vi "SP SP - get ctrl.vi"(8 "error in (no error)":errorcluster, 10 "subpanel":string, 11 "subsubpanel":string) -> (0 "error out":errorcluster, 2 "Boolean":bool, 3 "VI out":refnum<vi>)   [LabVIEW 2020, in "ui-testing.lvlib"]
uses:
  ui-testing.lvlib
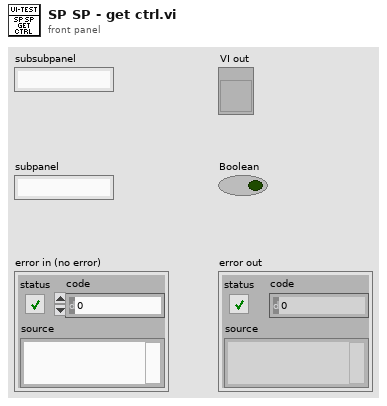
[diagram p1: front panel]
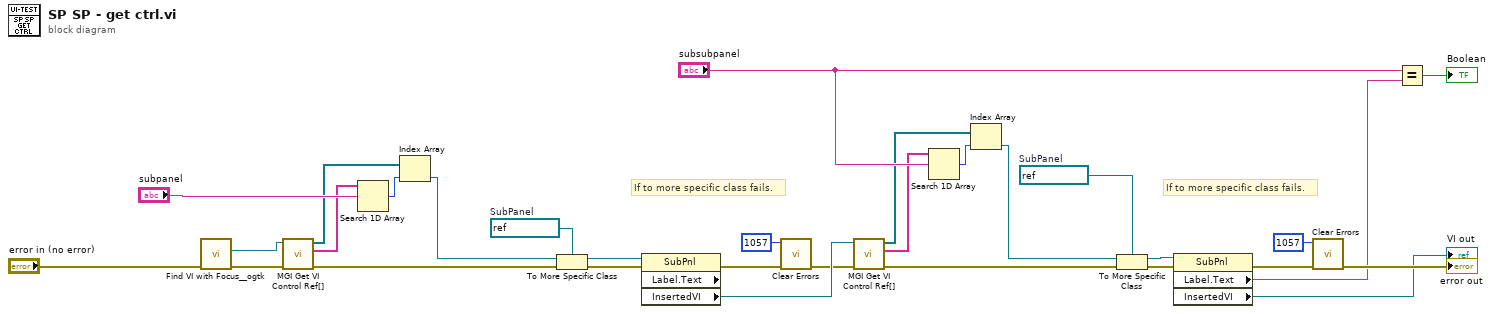
[diagram p0: block diagram]
diagram:
  w15 = refnum<vi> refnum  # SubPanel
  w11 = refnum<vi> refnum  # SubPanel
  # "If to more specific class fails."
  # "If to more specific class fails."
  n1 = call <userlib>:"Find VI with Focus__ogtk.vi"("error in"="error in (no error)") -> ("error out"=w6:errorcluster, "VI with Focus"=w5:refnum<vi>)  [unwired: 6 in, 3 out]
  n2 = call <userlib>:"MGI Get VI Control Ref[].vi"("error in"=w6, "VI (Caller)"=w5) -> ("error out"=w13:errorcluster, "Control Label Chain[i]"=w2:string[], "Control[i]"=w3:refnum<vi>[])  [unwired: 6 in, 1 out]
  n3 = Search 1D Array(1D array=w2, element="subpanel") -> (index of element=w4:i32)  [unwired: 1 in]
  n4 = Index Array(array=w3, index=w4) -> (element=w14:refnum<vi>)
  n5 = To More Specific Class(target class=w11, reference=w14, error in=w13) -> (specific class reference=w12:refnum<vi>, error out=w10:errorcluster)
  n6 = property class="SubPnl" props=["Label", "Text", "InsertedVI"](reference=w12, error in=w10) -> (error out=w8:errorcluster, "InsertedVI"=w30:refnum<vi>)  [unwired: 2 out]
  n7 = call <vilib>:"Clear Errors.vi"("error in (no error)"=w8, "specific error code to clear (0: all)"=1057) -> ("error out"=w27:errorcluster)  [unwired: 4 in, 1 out]
  n8 = call <userlib>:"MGI Get VI Control Ref[].vi"("error in"=w27, "VI (Caller)"=w30) -> ("error out"=w28:errorcluster, "Control Label Chain[i]"=w24:string[], "Control[i]"=w25:refnum<vi>[])  [unwired: 6 in, 1 out]
  n9 = Search 1D Array(1D array=w24, element="subsubpanel") -> (index of element=w26:i32)  [unwired: 1 in]
  n10 = Index Array(array=w25, index=w26) -> (element=w29:refnum<vi>)
  n11 = To More Specific Class(target class=w15, reference=w29, error in=w28) -> (specific class reference=w16:refnum<vi>, error out=w17:errorcluster)
  n12 = property class="SubPnl"(reference=w16, error in=w17) -> (error out=w21:errorcluster, "Label.Text"=w18:string, "InsertedVI"=→"VI out":refnum<vi>)  [unwired: 1 out]
  n13 = call <vilib>:"Clear Errors.vi"("error in (no error)"=w21, "specific error code to clear (0: all)"=1057) -> ("error out"=→"error out":errorcluster)  [unwired: 4 in, 1 out]
  n14 = Equal?(x="subsubpanel", y=w18) -> (x = y?=→"Boolean":bool)
